vi "Dialogue Window-3 button.vi"(6 "Caption-Left button (Cancel)":string, 7 "Colour":u32(colorbox)=16777225, 8 "error in (no error)":errorcluster, 9 "Caption-Middle button":string, 10 "Caption-Right button (OK)":string, 11 "Message string":string) -> (0 "error out":errorcluster, 1 "Cancelled (Left button pressed)":bool, 3 "Button pressed":T1)   [LabVIEW 2020]
doc: "Use this template to create a dialog box with event handling."
uses:
  Typedefs/Button Pressed.ctl
  <vilib>/Utility/miscctls.llb/LVPointTypeDef.ctl
  Global Variables/General Globals.vi
panel:
  in  "Middle Button":bool
  in  "Left Button":bool
  in  "Rigth Button":bool
  out "Message":string
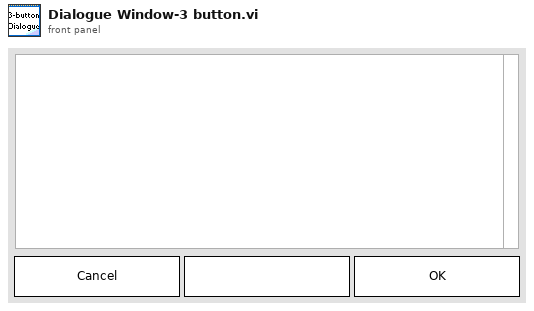
[diagram p1: front panel]
types:
  T1 = typedef "Button Pressed.ctl" = enum16{"Left button", "Middle button", "Right button"}
  T2 = typedef "LVPointTypeDef.ctl" = cluster{"Horizontal":i16, "Vertical":i16}
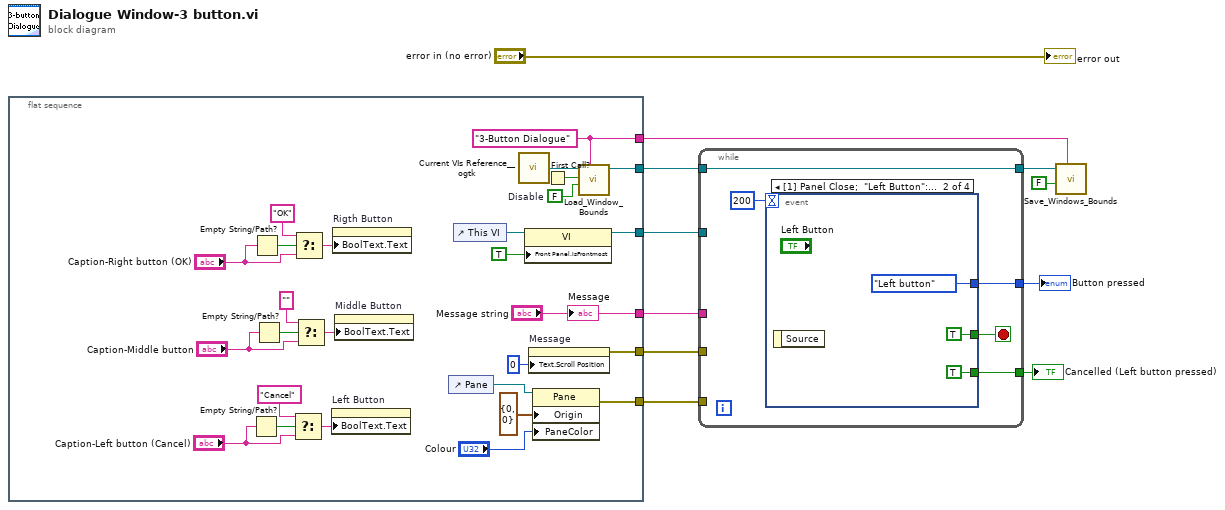
[diagram p0: block diagram]
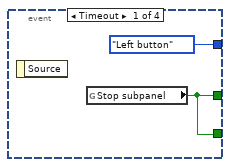
[diagram p2: hidden frame]
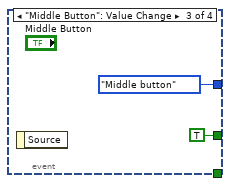
[diagram p3: hidden frame]
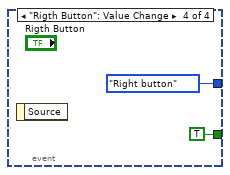
[diagram p4: hidden frame]
diagram:
  n1 = flat-sequence {
    tunnel: ["Message string"] -> w11
    tunnel: [w36] -> w10
    tunnel: [w33] -> w9
    tunnel: [w31] -> w8
    tunnel: [w26] -> w6
    tunnel: [w25] -> w4
    frame #0 {
      w27 = FALSE  # Disable
      w26 = "3-Button Dialogue" ("Window Name (i.e. Key)")
      n2 = Empty String/Path?(string/path="Caption-Left button (Cancel)") -> (empty?=w19:bool)
      n3 = Empty String/Path?(string/path="Caption-Right button (OK)") -> (empty?=w23:bool)
      n4 = Empty String/Path?(string/path="Caption-Middle button") -> (empty?=w13:bool)
      n5 = Select(t="Cancel", s=w19, f="Caption-Left button (Cancel)") -> (s? t:f=w18:string)
      n6 = Select(t="OK", s=w23, f="Caption-Right button (OK)") -> (s? t:f=w21:string)
      n7 = Select(t="", s=w13, f="Caption-Middle button") -> (s? t:f=w14:string)
      n8 = property on="Left Button" class="Bool"("BoolText.Text"=w18) -> ()  [unwired: 2 in, 2 out]
      n9 = property on="Rigth Button" class="Bool"("BoolText.Text"=w21) -> ()  [unwired: 2 in, 2 out]
      n10 = property on="Middle Button" class="Bool"("BoolText.Text"=w14) -> ()  [unwired: 2 in, 2 out]
      n11 = control-ref of="Pane"() -> (w30:refnum<vi>)
      n12 = control-ref of="This VI"() -> (w34:refnum<vi>)
      n13 = call <userlib>:"Current VIs Reference__ogtk.vi"() -> ("Current VI's reference"=w29:refnum<vi>)  [unwired: 5 in]
      n14 = property on="Property Node" class="VI"(reference=w34, "Front Panel.IsFrontmost"=TRUE ("Front Panel Window:Is Frontmost")) -> (reference out=w33:refnum<vi>)  [unwired: 1 in, 1 out]
      n15 = property on="Message" class="Str"("Text.Scroll Position"=u32 0) -> (error out=w36:errorcluster)  [unwired: 2 in, 1 out]
      n16 = property class="Pane"(reference=w30, "Origin"=T2 {"Horizontal"=0, "Vertical"=0}, "PaneColor"="Colour") -> (error out=w31:errorcluster)  [unwired: 1 in, 1 out]
      n17 = First Call?() -> (First Call?: T/F=w28:bool)
      n18 = call "Load_Window_Bounds.vi"("Window Name (i.e. Key)"=w26, "Disable"=w27, "First Call"=w28, "Window VI's Ref"=w29) -> ("reference out"=w25:refnum<vi>)  [unwired: 4 in, 3 out]
      "Message" <- "Message string"
    }
  }
  n19 = while {
    tunnel: w11 -> [_]
    tunnel: w10 -> [_]
    tunnel: w8 -> [_]
    tunnel: w9 -> [_]
    tunnel: [w41] -> w7
    tunnel: w4 -> [w40]
    tunnel: [w40] -> w3
    tunnel: [w39] -> w1
    stop <- w43 stop-if-true
    n20 = event shown="[1] Panel Close;  \"Left Button\": Value Change" {
      selector: _ -> [_ _ _ _]
      dyn-events: _ -> [_ _ _ _]
      timeout: 200 -> [_ _ _ _]
      tunnel: [w45 TRUE ("Stop?") TRUE ("Stop?") TRUE ("Stop?")] -> w43
      tunnel: [w45 TRUE ("Stop subpanel") _ _] -> w41
      tunnel: [Button_Pressed."Left button" ("Button pressed") Button_Pressed."Left button" ("Button pressed") Button_Pressed."Middle button" ("Button pressed") Button_Pressed."Right button" ("Button pressed")] -> w39
      event Timeout {
        n21 = event-data() -> ()  [unwired: 1 in, 1 out]
        n22 = global read "General Globals.vi" "Stop subpanel"() -> (w45:bool)
      }
      event Panel Close; "Left Button": Value Change {
        n23 = event-data() -> ()  [unwired: 1 in, 1 out]
      }
      event "Middle Button": Value Change {
        n24 = event-data() -> ()  [unwired: 1 in, 1 out]
      }
      event "Rigth Button": Value Change {
        n25 = event-data() -> ()  [unwired: 1 in, 1 out]
      }
    }
  }
  "Cancelled (Left button pressed)" <- w7
  "Button pressed" <- w1
  n26 = call "Save_Windows_Bounds.vi"("Window Name (i.e. Key)"=w6, "Front Panel Window:Open"=FALSE, "Window VI's Ref"=w3) -> ()  [unwired: 8 in, 1 out]
  "error out" <- "error in (no error)"
